vi "Read CAN Frames.vi"(8 "error in (no error)":errorcluster, 9 "Length (all)":i32=-1, 10 "Offset":i32, 11 "BLF File In":refnum<class "Read Write BLF.lvclass">) -> (0 "error out":errorcluster, 1 "CAN Channels":u16[](array[numeric]), 2 "CAN Frames":T1[](array[typedef]) {"type" items=["CAN Data"=0, "CAN Remote"=1, "CAN Bus Error"=2, "CAN 2.0 Data"=8, "CAN FD Data"=16, "CAN FD+BRS Data"=24, "J1939 Data"=192, "Delay"=224, "Log Trigger"=225, "Start Trigger"=226]; "payload" format="%x"; "timestamp" format="%<%.7X\n%x>T"; "identifier" format="%x"}, 3 "BLF File Out":refnum<class "Read Write BLF.lvclass">)   [LabVIEW 2015, in "Read Write BLF.lvclass"]
doc: "This VI will read <B>CAN Frames</B> from a BLF file. Optionally enter the <B>Offset</B> and <B>Length</B> which defaults to all. This will read the set number of Objects which might not correspond to the same number of frames.\n\n-------------\nBrian Hoover (Hooovahh)"
uses:
  Read Write BLF.lvclass
  Controls/Cluster - CAN Frame.ctl
  Controls/Enum - CAN Data Type.ctl
  Read Write BLF.lvclass/Read Write BLF.ctl
  Controls/Enum - Read Object Types.ctl
  SubVIs/GetBinlogdllpath.vi
  <vilib>/Utility/error.llb/Error Cluster From Error Code.vi
  <vilib>/Utility/libraryn.llb/Check if File or Folder Exists.vi
  <vilib>/Utility/file.llb/Application Directory.vi
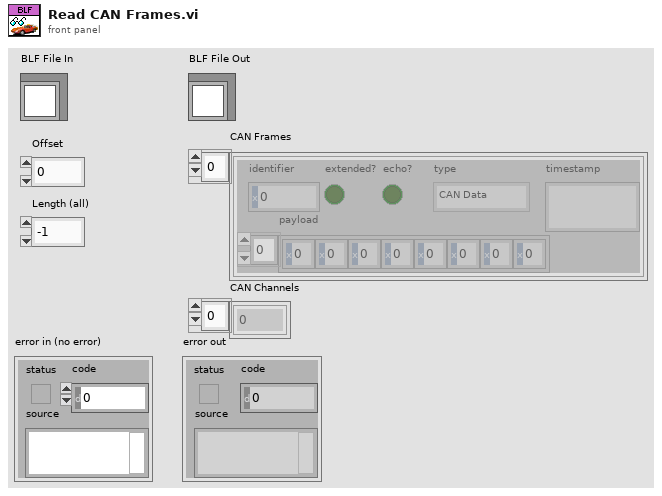
[diagram p1: front panel]
types:
  T1 = typedef "Read Write BLF.lvclass/Cluster - CAN Frame.ctl" = cluster{"timestamp":timestamp, "payload":u8[], "identifier":u32, "extended?":bool, "echo?":bool, "type":T2}
  T2 = typedef "Read Write BLF.lvclass/Enum - CAN Data Type.ctl" = u8
  T3 = typedef "Read Write BLF.lvclass/Enum - Read Object Types.ctl" = enum32{"UNKNOWN", "CAN_MESSAGE", "CAN_ERROR", "CAN_OVERLOAD", "CAN_STATISTIC", "APP_TRIGGER", "ENV_INTEGER", "ENV_DOUBLE", "ENV_STRING", "ENV_DATA", "LOG_CONTAINER", "LIN_MESSAGE", "LIN_CRC_ERROR", "LIN_DLC_INFO", "LIN_RCV_ERROR", "LIN_SND_ERROR", "LIN_SLV_TIMEOUT", "LIN_SCHED_MODCH", "LIN_SYN_ERROR", "LIN_BAUDRATE", "LIN_SLEEP", "LIN_WAKEUP", "MOST_SPY", "MOST_CTRL", "MOST_LIGHTLOCK", "MOST_STATISTIC", "reserved_1", "reserved_2", "reserved_3", "FLEXRAY_DATA", "FLEXRAY_SYNC", "CAN_DRIVER_ERROR", "MOST_PKT", "MOST_PKT2", "MOST_HWMODE", "MOST_REG", "MOST_GENREG", "MOST_NETSTATE", "MOST_DATALOST", "MOST_TRIGGER", "FLEXRAY_CYCLE", "FLEXRAY_MESSAGE", "LIN_CHECKSUM_INFO", "LIN_SPIKE_EVENT", "CAN_DRIVER_SYNC", "FLEXRAY_STATUS", "GPS_EVENT", "FR_ERROR", "FR_STATUS", "FR_STARTCYCLE", "FR_RCVMESSAGE", "REALTIMECLOCK", "AVAILABLE2", "AVAILABLE3", "LIN_STATISTIC", "J1708_MESSAGE", "J1708_VIRTUAL_MSG", "LIN_MESSAGE2", "LIN_SND_ERROR2", "LIN_SYN_ERROR2", "LIN_CRC_ERROR2", "LIN_RCV_ERROR2", "LIN_WAKEUP2", "LIN_SPIKE_EVENT2", "LIN_LONG_DOM_SIG", "APP_TEXT", "FR_RCVMESSAGE_EX", "MOST_STATISTICEX", "MOST_TXLIGHT", "MOST_ALLOCTAB", "MOST_STRESS", "ETHERNET_FRAME", "SYS_VARIABLE", "CAN_ERROR_EXT", "CAN_DRIVER_ERROR_EXT", "LIN_LONG_DOM_SIG2", "MOST_150_MESSAGE", "MOST_150_PKT", "MOST_ETHERNET_PKT", "MOST_150_MESSAGE_FRAGMENT", "MOST_150_PKT_FRAGMENT", "MOST_ETHERNET_PKT_FRAGMENT", "MOST_SYSTEM_EVENT", "MOST_150_ALLOCTAB", "MOST_50_MESSAGE", "MOST_50_PKT", "CAN_MESSAGE2", "LIN_UNEXPECTED_WAKEUP", "LIN_SHORT_OR_SLOW_RESPONSE", "LIN_DISTURBANCE_EVENT", "SERIAL_EVENT", "OVERRUN_ERROR", "EVENT_COMMENT", "WLAN_FRAME", "WLAN_STATISTIC", "MOST_ECL", "GLOBAL_MARKER", "AFDX_FRAME", "AFDX_STATISTIC", "KLINE_STATUSEVENT", "CAN_FD_MESSAGE", "CAN_FD_MESSAGE_64", "ETHERNET_RX_ERROR", "ETHERNET_STATUS", "CAN_FD_ERROR_64", "LIN_SHORT_OR_SLOW_RESPONSE2", "AFDX_STATUS", "AFDX_BUS_STATISTIC"}
  T4 = typedef "Read Write BLF.lvclass/Cluster - mHeaderBase.ctl" = cluster{"mSignature":u32, "mHeaderSize":u16, "mHeaderVersion":u16, "mObjectSize":u32, "Object Type":T3}
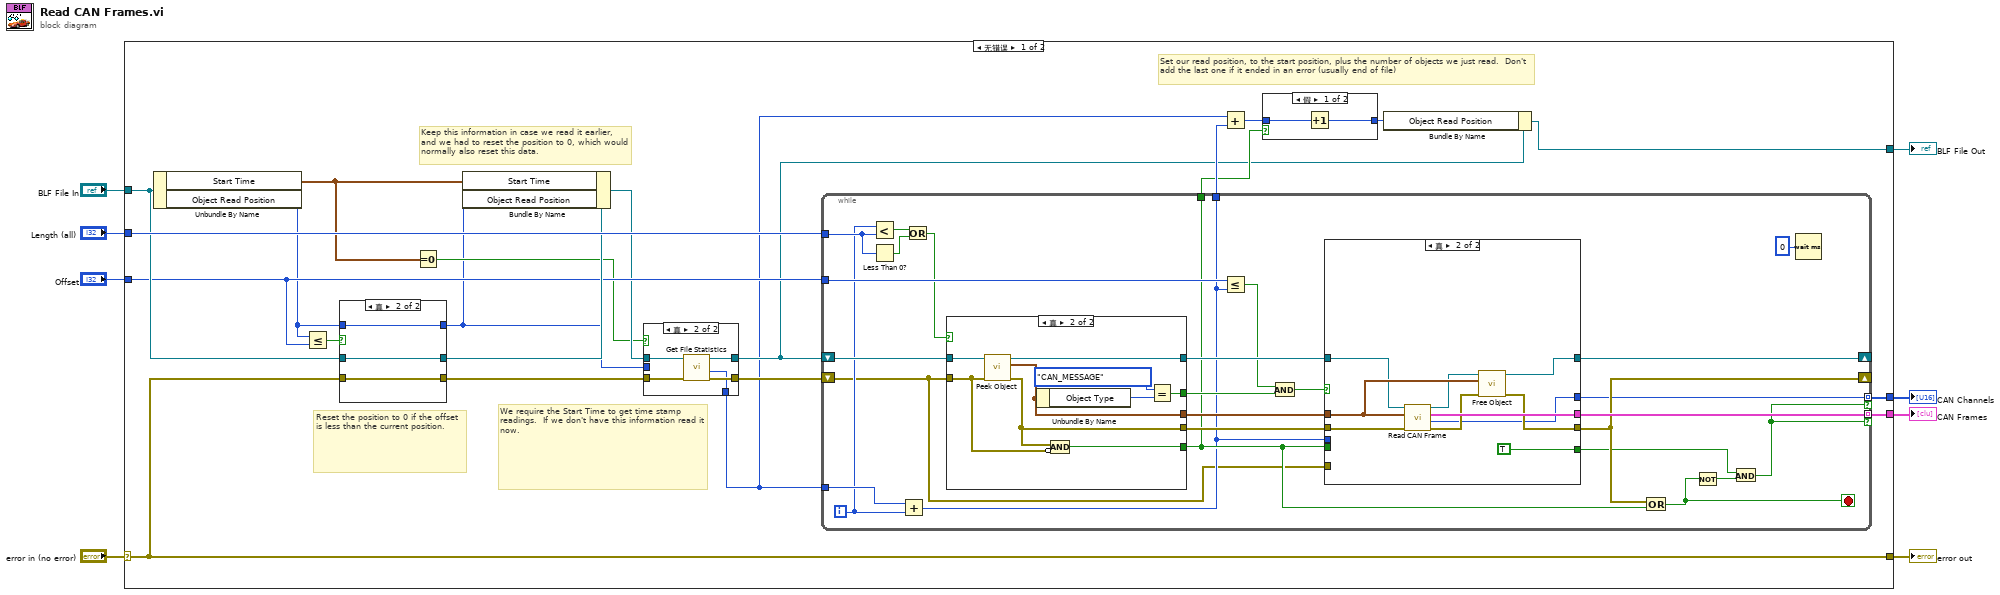
[diagram p0: block diagram]
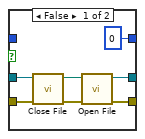
[diagram p3: hidden frame]
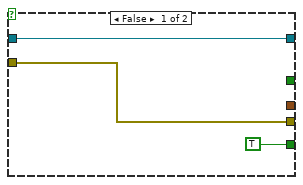
[diagram p5: hidden frame]
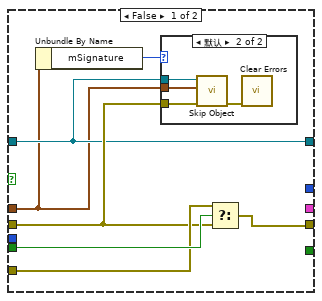
[diagram p6: hidden frame]
diagram:
  n1 = case shown="无错误" "error in (no error)" {
    selector: "error in (no error)" -> [w22 w112]
    tunnel: [w22 w112] -> w7
    tunnel: [w28 w111] -> w5
    tunnel: "BLF File In" -> [w23 w111]
    tunnel: [w30 _] -> w4
    tunnel: "Length (all)" -> [w29 _]
    tunnel: "Offset" -> [w18 _]
    tunnel: [w9 _] -> w1
    frame No Error {
      # "Set our read position, to the start position, plus the number of objects we just read.  Don't add the last one if it ended in an error (usually end of file)"
      # "We require the Start Time to get time stamp readings.  If we don't have this information read it now."
      # "Keep this information in case we read it earlier, and we had to reset the position to 0, which would normally also reset this data."
      # "Reset the position to 0 if the offset is less than the current position."
      n2 = Unbundle By Name(w23) -> ("Start Time"=w10:timestamp, "Object Read Position"=w14:u32)
      n3 = Less Or Equal?(x=w14, y=w18) -> (x <= y?=w17:bool)
      n4 = case shown="真" w17 {
        tunnel: [w43 w48] -> w20
        tunnel: [w42 w47] -> w21
        tunnel: w23 -> [w41 w48]
        tunnel: w22 -> [w40 w47]
        tunnel: w14 -> [_ w46]
        tunnel: [u32 0 ("Object Read Position") w46] -> w13
        frame False {
          n5 = call "Close File.vi"("error in (no error)"=w40, "BLF File"=w41) -> ("error out"=w45:errorcluster, "BLF Path"=w44:path)  [unwired: 8 in]
          n6 = call "Open File.vi"("error in (no error)"=w45, "Log Path"=w44) -> ("error out"=w42:errorcluster, "BLF File"=w43:refnum<class "Read Write BLF.lvclass">)  [unwired: 8 in]
        }
        frame True {
        }
      }
      n7 = Equal To 0?(x=w10) -> (x = 0?=w15:bool)
      n8 = Bundle By Name(cluster=w20, "Start Time"=w10, "Object Read Position"=w13) -> (w16:refnum<class "Read Write BLF.lvclass">)
      n9 = case shown="真" w15 {
        tunnel: w21 -> [w32 w38]
        tunnel: w16 -> [w33 w37]
        tunnel: [w33 w35] -> w12
        tunnel: [w32 w36] -> w19
        tunnel: [w31 w34] -> w11
        tunnel: w13 -> [w31 _]
        frame False {
        }
        frame True {
          n10 = call "Get File Statistics.vi"("error in (no error)"=w38, "Read Write BLF in"=w37) -> ("error out"=w36:errorcluster, "Objecs Read Position"=w34:u32, "Read Write BLF out"=w35:refnum<class "Read Write BLF.lvclass">)  [unwired: 3 in, 4 out]
        }
      }
      n11 = while {
        shift-right: [w73] -> _
        shift-left: w19 -> [w54]
        shift-right: [w75] -> _
        shift-left: w12 -> [w70]
        tunnel: [w77] -> w30 mode=indexing if=w52
        tunnel: w29 -> [w66]
        tunnel: w18 -> [w63]
        tunnel: [w58] -> w27
        tunnel: [w59] -> w25
        tunnel: w11 -> [w57]
        tunnel: [w53] -> w9 mode=indexing if=w52
        i -> [w56]
        stop <- w72 stop-if-true
        n12 = Less?(x=w56, y=w66) -> (x < y?=w65:bool)
        n13 = Less Than 0?(x=w66) -> (x < 0?=w64:bool)
        n14 = Add(x=w57, y=w56) -> (x+y=w58:u32)
        n15 = Or(x=w65, y=w64) -> (x .or. y?=w55:bool)
        n16 = case shown="真" w55 {
          tunnel: [w80 w89] -> w76
          tunnel: [w79 w87] -> w74
          tunnel: w54 -> [w79 w86]
          tunnel: [_ w85] -> w71
          tunnel: w70 -> [w80 w84]
          tunnel: [_ w83] -> w69
          tunnel: [TRUE w81] -> w59
          frame False {
          }
          frame True {
            n17 = call "Peek Object.vi"("error in (no error)"=w86, "BLF File In"=w84) -> ("error out"=w87:errorcluster, "Header Read"=w85:T4, "BLF File Out"=w89:refnum<class "Read Write BLF.lvclass">)  [unwired: 7 in]
            n18 = Unbundle By Name(w85) -> ("Object Type"=w88:T3)
            n19 = Compound Arithmetic op=AND(w87, invert w86) -> (w81:bool)
            n20 = Equal?(x=Enum_-_Read_Object_Types."CAN_MESSAGE", y=w88) -> (x = y?=w83:bool)
          }
        }
        n21 = Less Or Equal?(x=w63, y=w58) -> (x <= y?=w62:bool)
        n22 = Compound Arithmetic op=AND(w62, w69) -> (w68:bool)
        n23 = case shown="真" w68 {
          tunnel: [_ w110] -> w77
          tunnel: w76 -> [w92 w104]
          tunnel: [w92 w106] -> w75
          tunnel: w74 -> [w93 w109]
          tunnel: [w94 w107] -> w73
          tunnel: w71 -> [w91 w108]
          tunnel: w59 -> [w96 _]
          tunnel: w54 -> [w95 _]
          tunnel: w58 -> [_ _]
          tunnel: [_ TRUE] -> w60
          tunnel: [_ w101] -> w53
          frame False {
            n24 = Unbundle By Name(w91) -> ("mSignature"=w90:u32)
            n25 = case shown="默认" w90 {
              tunnel: w93 -> [_ w100]
              tunnel: w92 -> [_ w98]
              tunnel: w91 -> [_ w97]
              frame 0 {
              }
              frame Default {
                n26 = call "Skip Object.vi"("error in (no error)"=w100, "Header"=w97, "BLF File In"=w98) -> ("error out"=w99:errorcluster)  [unwired: 7 in, 1 out]
                n27 = call <vilib>:"Clear Errors.vi"("error in (no error)"=w99) -> ()  [unwired: 5 in, 2 out]
              }
            }
            n28 = Select(t=w95, s=w96, f=w93) -> (s? t:f=w94:errorcluster)
          }
          frame True {
            n29 = call "Read CAN Frame.vi"("error in (no error)"=w109, "Header Read"=w108, "BLF File In"=w104) -> ("error out"=w105:errorcluster, "CAN Channel"=w101:u16, "CAN Frame"=w110:T1, "BLF File Out"=w103:refnum<class "Read Write BLF.lvclass">)  [unwired: 5 in]
            n30 = call "Free Object.vi"("error in (no error)"=w105, "Header"=w108, "BLF File In"=w103) -> ("error out"=w107:errorcluster, "BLF File Out"=w106:refnum<class "Read Write BLF.lvclass">)  [unwired: 7 in]
          }
        }
        n31 = Compound Arithmetic op=OR(w73, w59) -> (w72:bool)
        n32 = Not(x=w72) -> (.not. x?=w67:bool)
        n33 = And(x=w60, y=w67) -> (x .and. y?=w52:bool)
        n34 = Wait (ms)(milliseconds to wait=u32 0) -> ()  [unwired: 1 out]
      }
      n35 = Add(x=w11, y=w27) -> (x+y=w26:u32)
      n36 = case shown="假" w25 {
        tunnel: w26 -> [w50 w51]
        tunnel: [w49 w51] -> w24
        frame False {
          n37 = Increment(x=w50) -> (x+1=w49:u32)
        }
        frame True {
        }
      }
      n38 = Bundle By Name(cluster=w12, "Object Read Position"=w24) -> (w28:refnum<class "Read Write BLF.lvclass">)
    }
    frame Error {
    }
  }
  "error out" <- w7
  "BLF File Out" <- w5
  "CAN Frames" <- w4
  "CAN Channels" <- w1
